vi "DSF.Engine.Memory.Pointer.VS Channels.Valid.vi"(8 "error in (no error)":errorcluster, 11 "VS Channels Pointer in":refnum<class "DSF.Engine.Memory.Pointer.VS Channels.lvclass">) -> (0 "error out":errorcluster, 3 "VS Channels Pointer out":refnum<class "DSF.Engine.Memory.Pointer.VS Channels.lvclass">)   [LabVIEW 2016, in "DSF.Engine.lvlib" / "DSF.Engine.Memory.Pointer.VS Channels.lvclass"]
uses:
  DSF.Engine.Memory.Pointer.VS Channels.lvclass
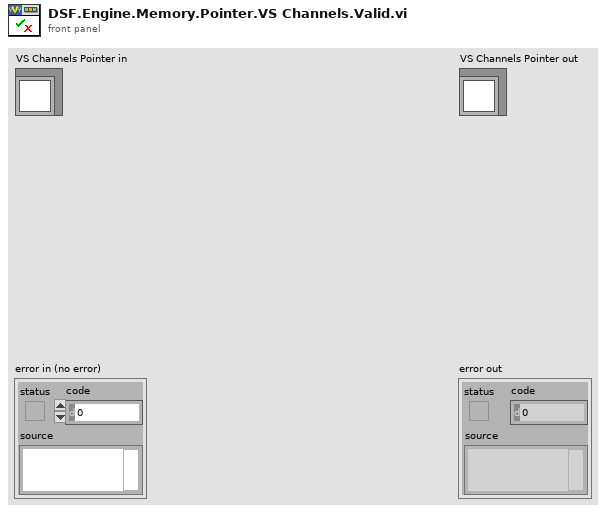
[diagram p1: front panel]
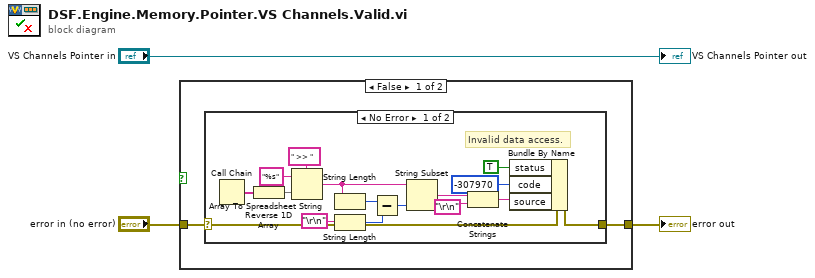
[diagram p0: block diagram]
diagram:
  n1 = case shown="False" w4 {
    tunnel: "error in (no error)" -> [w6 w24]
    tunnel: [w5 w24] -> w3
    frame False {
      n2 = case shown="No Error" w6 {
        selector: w6 -> [w19 w23]
        tunnel: [w22 w23] -> w5
        frame No Error {
          # "Invalid data access."
          n3 = Call Chain() -> (call chain=w8:string[])
          n4 = Reverse 1D Array(array=w8) -> (reversed array=w15:string[])
          n5 = Array To Spreadsheet String(delimiter (Tab)=" >> ", array=w15, 3:"%s" ("format string")) -> (spreadsheet string=w16:string)
          n6 = String Length(string=w16) -> (length=w14:i32)
          n7 = String Length(string="\r\n") -> (length=w18:i32)
          n8 = Subtract(x=w14, y=w18) -> (x-y=w13:i32)
          n9 = String Subset(string=w16, length (rest)=w13) -> (substring=w9:string)  [unwired: 1 out]
          n10 = Concatenate Strings(w9, "\r\n") -> (w7:string)
          n11 = Bundle By Name(cluster=w19, "status"=TRUE, "code"=-307970, "source"=w7) -> (w22:errorcluster)
        }
        frame Error {
          # "Leave existing error."
        }
      }
    }
    frame True {
    }
  }
  "error out" <- w3
  "VS Channels Pointer out" <- "VS Channels Pointer in"
